vi "Test Preview Element.vi"() -> ()   [LabVIEW 2013]
uses:
  ByteFIFO/ByteFIFO.lvclass
  VariantBuffer/VariantBuffer.lvclass
panel:
  out "bytes 2":u8[](array[numeric]) format="%02x"
  out "bytes":u8[](array[numeric]) format="%02x"
  out "read elements ordering (index) - buffer full":bool
  out "read elements ordering (array) - buffer full":bool
  out "read element ordering (index) - buffer not full":bool
  out "read element ordering (array) - buffer not full":bool
  out "previewed all elements - not full, not empty":bool
  out "previewed elements at all indices":bool
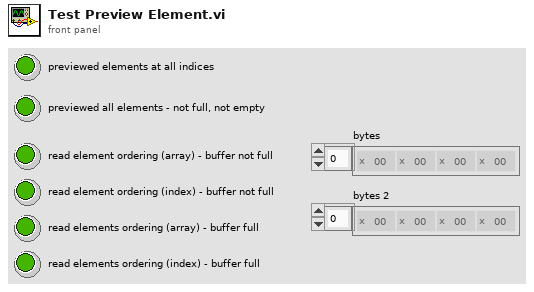
[diagram p1: front panel]
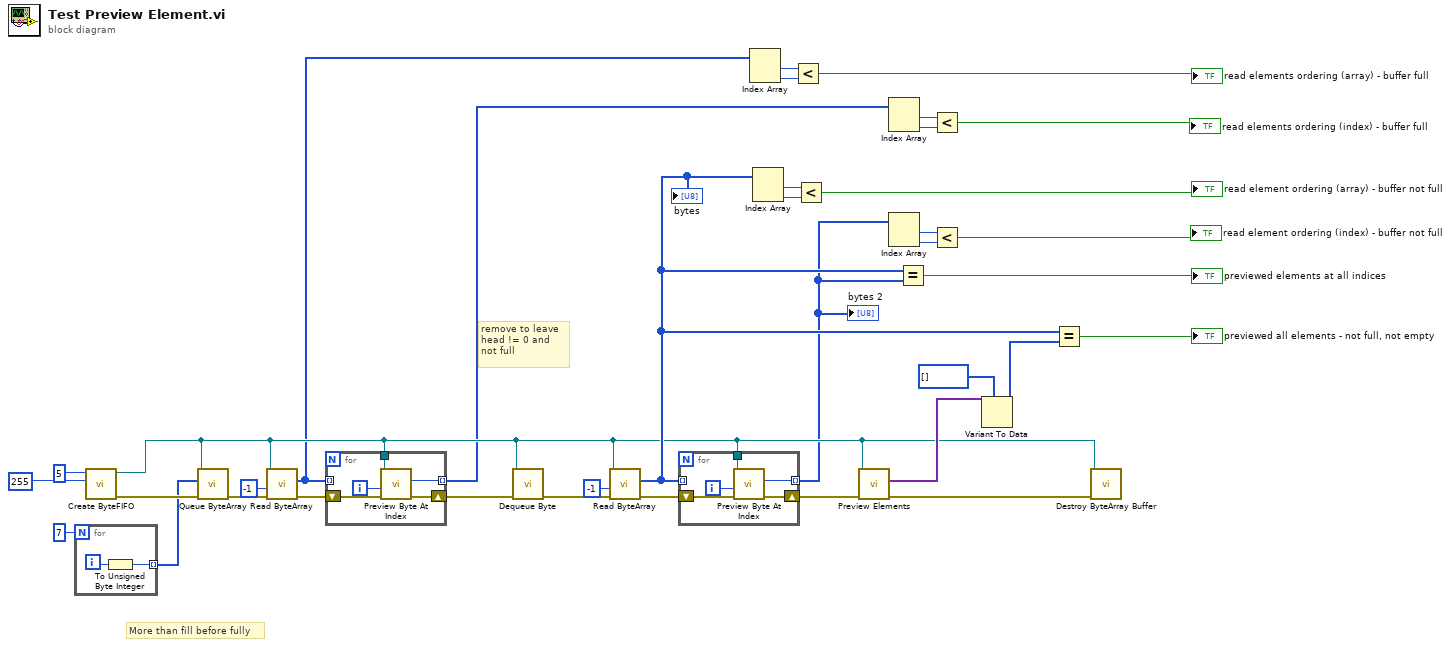
[diagram p0: block diagram]
diagram:
  # "remove to leave \nhead != 0 and\nnot full"
  # "More than fill before fully"
  n1 = for {
    N: 7 -> [_]
    tunnel: [w37] -> w32 mode=indexing
    i -> [w38]
    n2 = To Unsigned Byte Integer(number=w38) -> (unsigned 8bit integer=w37:u8)
  }
  n3 = call "Create ByteFIFO.vi"("default value"=u8 255, "bufSize"=5) -> ("error out"=w34:errorcluster, "Buffer"=w7:refnum<data-value>)  [unwired: 8 in]
  n4 = call "Queue ByteArray.vi"("error in"=w34, "bytes"=w32, "Buffer"=w7) -> ("error out"=w13:errorcluster)  [unwired: 6 in, 2 out]
  n5 = call "Read ByteArray.vi"("error in"=w13, "count (-1: all)"=-1, "Buffer"=w7) -> ("error out"=w9:errorcluster, "bytes"=w6:u8[])  [unwired: 6 in, 1 out]
  n6 = for {
    tunnel: w7 -> [w41]
    tunnel: [w40] -> w3 mode=indexing
    shift-right: [w39] -> w8
    shift-left: w9 -> [w43]
    tunnel: w6 -> [_] mode=indexing
    i -> [w42]
    n7 = call "Preview Byte At Index.vi"("error in (no error)"=w43, "index (-1: last)"=w42, "ByteFIFO"=w41) -> ("error out"=w39:errorcluster, "byte"=w40:u8)  [unwired: 5 in, 2 out]
  }
  n8 = call "Dequeue Byte.vi"("error in"=w8, "Buffer"=w7) -> ("error out"=w31:errorcluster)  [unwired: 6 in, 3 out]
  n9 = call "Read ByteArray.vi"("error in"=w31, "count (-1: all)"=-1, "Buffer"=w7) -> ("error out"=w30:errorcluster, "bytes"=w22:u8[])  [unwired: 6 in, 1 out]
  "bytes" <- w22
  n10 = for {
    tunnel: w7 -> [w46]
    tunnel: w22 -> [_] mode=indexing
    tunnel: [w45] -> w1 mode=indexing
    shift-right: [w44] -> w28
    shift-left: w30 -> [w48]
    i -> [w47]
    n11 = call "Preview Byte At Index.vi"("error in (no error)"=w48, "index (-1: last)"=w47, "ByteFIFO"=w46) -> ("error out"=w44:errorcluster, "byte"=w45:u8)  [unwired: 5 in, 2 out]
  }
  "bytes 2" <- w1
  n12 = Index Array(array=w6) -> (element #1=w11:u8, element #2=w12:u8)  [unwired: 2 in]
  n13 = Index Array(array=w22) -> (element #1=w21:u8, element #2=w20:u8)  [unwired: 2 in]
  n14 = Less?(x=w11, y=w12) -> (x < y?=→"read elements ordering (array) - buffer full":bool)
  n15 = Less?(x=w21, y=w20) -> (x < y?=→"read element ordering (array) - buffer not full":bool)
  n16 = call "Preview Elements.vi"("error in"=w28, "ByteBuffer in"=w7) -> ("error out"=w27:errorcluster, "elements"=w26:variant[])  [unwired: 7 in, 1 out]
  n17 = Index Array(array=w3) -> (element #1=w5:u8, element #2=w4:u8)  [unwired: 2 in]
  n18 = Index Array(array=w1) -> (element #1=w16:u8, element #2=w17:u8)  [unwired: 2 in]
  n19 = Equal?(x=w22, y=w1) -> (x = y?=→"previewed elements at all indices":bool)
  n20 = Less?(x=w5, y=w4) -> (x < y?=→"read elements ordering (index) - buffer full":bool)
  n21 = Less?(x=w16, y=w17) -> (x < y?=→"read element ordering (index) - buffer not full":bool)
  n22 = Variant To Data(type=u8[] [], Variant=w26) -> (data=w24:u8[])  [unwired: 1 in, 1 out]
  n23 = Equal?(x=w22, y=w24) -> (x = y?=→"previewed all elements - not full, not empty":bool)
  n24 = call "Destroy ByteArray Buffer.vi"("error in"=w27, "Buffer"=w7) -> ()  [unwired: 8 in, 2 out]
